vi "NT_LL_Get Persistent.vi"(8 "error in (no error)":errorcluster, 11 "topicHandle":u32) -> (0 "error out":errorcluster, 3 "Persistence":bool)   [LabVIEW 2025]
uses:
  ntcoreffi.dll
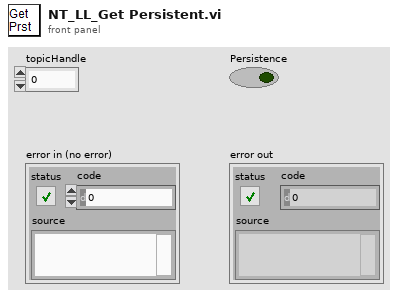
[diagram p1: front panel]
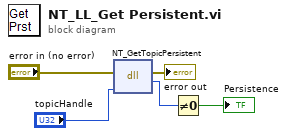
[diagram p0: block diagram]
diagram:
  n1 = dll-call lib="ntcoreffi.*" fn="NT_GetTopicPersistent"(error in="error in (no error)", "topicHandle"="topicHandle") -> (error out=→"error out":errorcluster, "value"=w3:u32)  [unwired: 3 in, 1 out]
  n2 = Not Equal To 0?(x=w3) -> (x != 0?=→"Persistence":bool)
